vi "open16.vi"(8 "error in (no error)":errorcluster, 10 "ppDb":dbl, 11 "filename":u32) -> (0 "error out":errorcluster, 2 "ppDb out":dbl, 3 "function return":i32)   [LabVIEW 2020, in "sqlite3.lvlib"]
uses:
  sqlite3.lvlib
  errstr.vi
  bin/sqlite3_64.dll
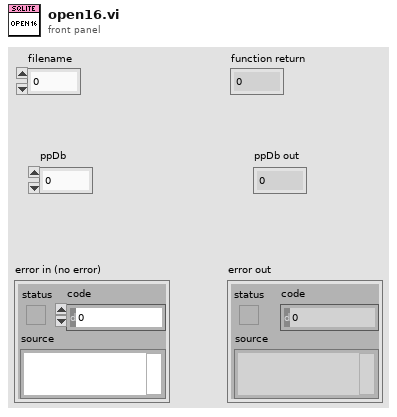
[diagram p1: front panel]
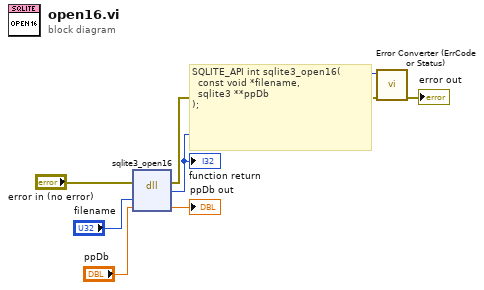
[diagram p0: block diagram]
diagram:
  # "SQLITE_API int sqlite3_open16(\n  const void *filename,   \n  sqlite3 **ppDb          \n);"
  n1 = dll-call lib="D:/Project/Labview-Projects/database-configuration/externals/sqlite3/Source/bin/sqlite3_*.*" fn="sqlite3_open16"(error in="error in (no error)", "filename"="filename", "ppDb"="ppDb") -> (error out=w2:errorcluster, w7:i32, "ppDb"=→"ppDb out":dbl)  [unwired: 3 in, 1 out]
  "function return" <- w7
  n2 = call "Error Converter (ErrCode or Status).vi"("error in (no error)"=w2, "error code"=w7) -> ("error out"=→"error out":errorcluster)  [unwired: 9 in]
